vi "DataTreeCtrlFM readData.vi"(8 "error in (no error)":errorcluster, 10 "dataName":string, 11 "TDMSAdv in":refnum<class "TDMSAdv.lvclass">) -> (0 "error out":errorcluster, 2 "signalData":waveform(sgl), 3 "TDMSAdv out":refnum<class "TDMSAdv.lvclass">)   [LabVIEW 2018, in "DataTreeCtrl.lvclass"]
uses:
  DataTreeCtrl.lvclass
  PublicSubVI/Class/FileManager/TDMSAdv.lvclass
  PublicSubVI/Class/FileManager/FM/ctl/_PC_Pub_FM fileReadFuncEnum.ctl
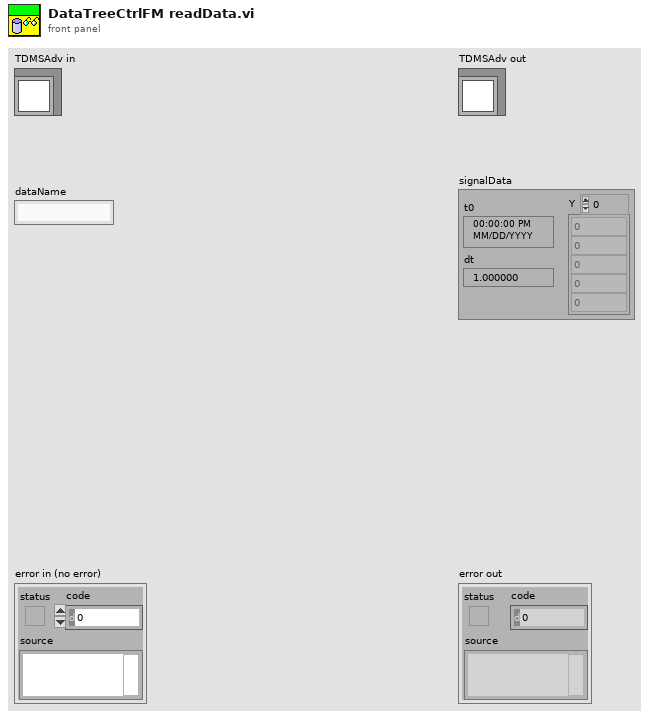
[diagram p1: front panel]
types:
  T1 = typedef "_PC_Pub_FM fileReadFuncEnum.ctl" = enum16{"getAllInfo", "getChromatogram", "getDataItems", "getTimeStamp", "getIdxData", "getIonization", "getRemark", "getAttrFormat"}
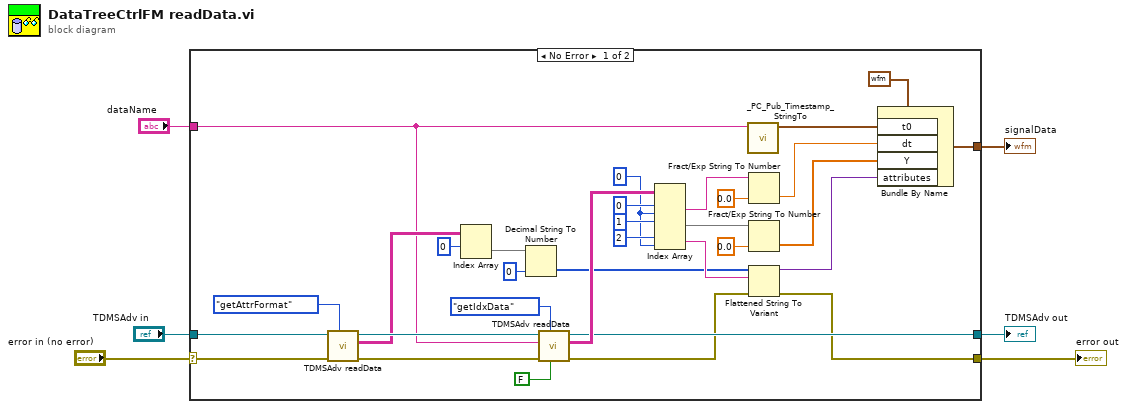
[diagram p0: block diagram]
diagram:
  n1 = case shown="No Error" "error in (no error)" {
    selector: "error in (no error)" -> [w11 w40]
    tunnel: "dataName" -> [w18 _]
    tunnel: [w8 w40] -> w4
    tunnel: [w13 _] -> w5
    tunnel: [w10 w39] -> w2
    tunnel: "TDMSAdv in" -> [w12 w39]
    frame No Error {
      w17 = 0 ("disabled index (col)")
      n2 = call "TDMSAdv readData.vi"("readEvent"=_PC_Pub_FM_fileReadFuncEnum."getAttrFormat", "error in (no error)"=w11, "TDMSAdv in"=w12) -> ("error out"=w33:errorcluster, "outputArr"=w34:string[][], "TDMSAdv out"=w36:refnum<class "TDMSAdv.lvclass">)  [unwired: 5 in, 1 out]
      n3 = Index Array(array=w34, index (row)=0) -> (element=w31:string[])  [unwired: 1 in]
      n4 = Decimal String To Number(string=w31, default (0L)=i16 0 ("default (0 I32)")) -> (number=w7:i16[])  [unwired: 1 in, 1 out]
      n5 = call "TDMSAdv readData.vi"("stringSplit? (T)"=FALSE, "readEvent"=_PC_Pub_FM_fileReadFuncEnum."getIdxData", "error in (no error)"=w33, "timeStamp"=w18, "TDMSAdv in"=w36) -> ("error out"=w9:errorcluster, "outputArr"=w27:string[][], "TDMSAdv out"=w10:refnum<class "TDMSAdv.lvclass">)  [unwired: 3 in, 1 out]
      n6 = Index Array(array=w27, index (row) #1=0 ("index (row)"), index (col) #1=w17, index (row) #2=1 ("index (row)"), index (row) #3=2 ("index (row)"), index (col) #3=w17) -> (element #1=w20:string, element #2=w19:string[], element #3=w16:string)  [unwired: 1 in]
      n7 = call "_PC_Pub_Timestamp_StringTo.vi"("Timestring"=w18) -> ("Timestamp"=w24:timestamp)  [unwired: 9 in, 1 out]
      n8 = Fract/Exp String To Number(string=w20, default (0 dbl)=0.0 ("default (0 DBL)")) -> (number=w22:dbl)  [unwired: 2 in, 1 out]
      n9 = Fract/Exp String To Number(string=w19, default (0 dbl)=sgl 0.0 ("default (0 DBL)")) -> (number=w21:sgl[])  [unwired: 2 in, 1 out]
      n10 = Flattened String To Variant(4:w9, 6:w16, 7:w7) -> (0:w8:errorcluster, 3:w14:variant)
      n11 = Bundle By Name(cluster=waveform(sgl) {"t0"=timestamp(0 s since 1904-01-01), "dt"=1.0, "Y"=[]} ("signal in"), "t0"=w24, "dt"=w22, "Y"=w21, "attributes"=w14) -> (w13:waveform(sgl))
    }
    frame Error {
    }
  }
  "error out" <- w4
  "signalData" <- w5
  "TDMSAdv out" <- w2
